vi "grabber tracking and stage files panel.vi"() -> ()   [LabVIEW 2010]
uses:
  tracking and stage files global.vi
panel:
  in  "stop":bool
  in  "auto-record":bool=TRUE
  in  "record":bool
  in  "record stage":bool=TRUE
  in  "record tracking":bool=TRUE
  in  "stub":string="lineName"
  in  "base directory":path
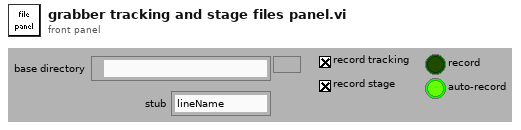
[diagram p1: front panel]
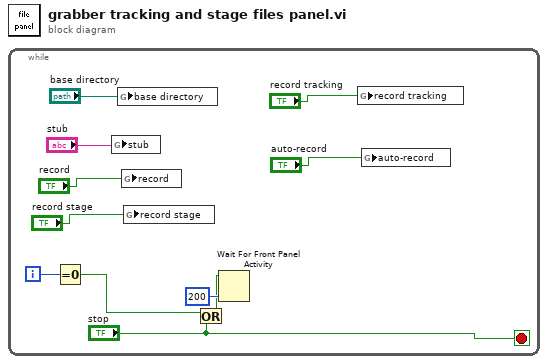
[diagram p0: block diagram]
diagram:
  n1 = while {
    i -> [w9]
    stop <- "stop" stop-if-true
    n2 = Equal To 0?(x=w9) -> (x = 0?=w7:bool)
    n3 = global write "tracking and stage files global.vi" "stub"("stub") -> ()
    n4 = global write "tracking and stage files global.vi" "base directory"("base directory") -> ()
    n5 = global write "tracking and stage files global.vi" "record"("record") -> ()
    n6 = global write "tracking and stage files global.vi" "record stage"("record stage") -> ()
    n7 = Or(x=w7, y="stop") -> (x .or. y?=w8:bool)
    n8 = Wait For Front Panel Activity(1:200 ("timeout ms (-1 never timeout)"), 3:w8) -> ()  [unwired: 1 in, 1 out]
    n9 = global write "tracking and stage files global.vi" "record tracking"("record tracking") -> ()
    n10 = global write "tracking and stage files global.vi" "auto-record"("auto-record") -> ()
  }
